vi "Labspec Load.vi"(8 "error in":errorcluster, 9 "Path":path, 11 "Automation Refnum In":refnum<k7>) -> (0 "error out":errorcluster, 1 "Data ID":i32, 3 "Automation Refnum Out":refnum<k7>)   [LabVIEW 2014]
panel:
  # "LICENSED MATERIALS – PROPERTY OF IBM\nCopyright IBM Corp. 2016,\nALL RIGHTS RESERVED"
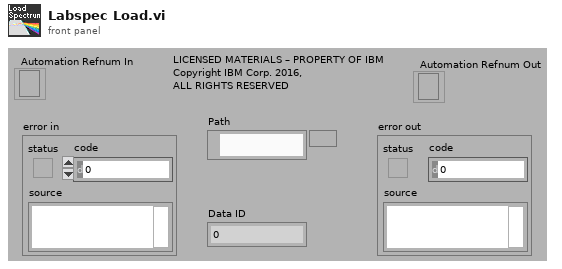
[diagram p1: front panel]
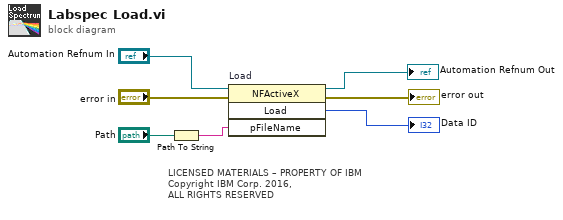
[diagram p0: block diagram]
diagram:
  # "LICENSED MATERIALS – PROPERTY OF IBM\nCopyright IBM Corp. 2016,\nALL RIGHTS RESERVED"
  n1 = Path To String(path="Path") -> (string=w5:string)
  n2 = invoke on="Load" class="NFActiveX" method="Load"(reference="Automation Refnum In", error in="error in", "pFileName"=w5) -> (reference out=→"Automation Refnum Out":refnum<k7>, error out=→"error out":errorcluster, "Load"=→"Data ID":i32)  [unwired: 1 in, 1 out]
